vi "CLD 14 Timer Application Solution.vi"() -> ()   [LabVIEW 2009]
doc: "CLD-Lösung 14. Dies ist ein Zustandsautomat in einer Queue. Als Queue wird ein Array verwendet. Der Timer wurde aus CLD-Übung 3 übernommen und angepasst.\n\nDie Timer-FGV läuft immer. Als Zeichen dafür, dass der Timer nicht \"aktiv\" ist, wird eine Zielzeit gleich null verwendet."
uses:
  CLD 14 State Machine Enum.ctl
  CLD 14 CSV file enum.ctl
  CLD 14 FGV Enum.ctl
panel:
  out "Zielzeit (s)":dbl
  out "Verstrichene Zeit (s)":dbl format="%#.2g"
  in  "Stopp":bool
  in  "Anhalten":bool
  in  "Abbrechen":bool
  in  "Starten":bool
  in  "Fehler (Eingang)":errorcluster
  out "Fehler (Ausgang)":errorcluster
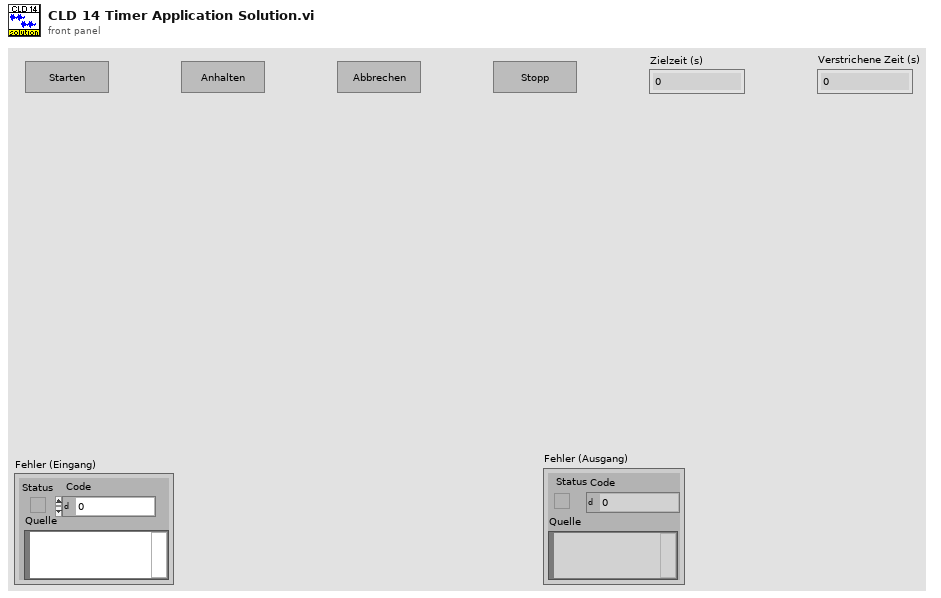
[diagram p1: front panel]
types:
  T1 = typedef "CLD 14 FGV Enum.ctl" = enum16{"Timer starten", "Zeit lesen", "Anhalten", "Fortsetzen"}
  T2 = typedef "CLD 14 State Machine Enum.ctl" = enum16{"Ruhezustand", "Initialisieren", "Zustand ausführen", "Zeit ändern", "Zeit prüfen", "Startzeit", "Anhalten", "Fortsetzen"}
  T3 = cluster{"Status":bool, "Code":i32, "Quelle":string}
  T4 = typedef "CLD 14 CSV file enum.ctl" = enum16{"CSV lesen", "CSV schreiben"}
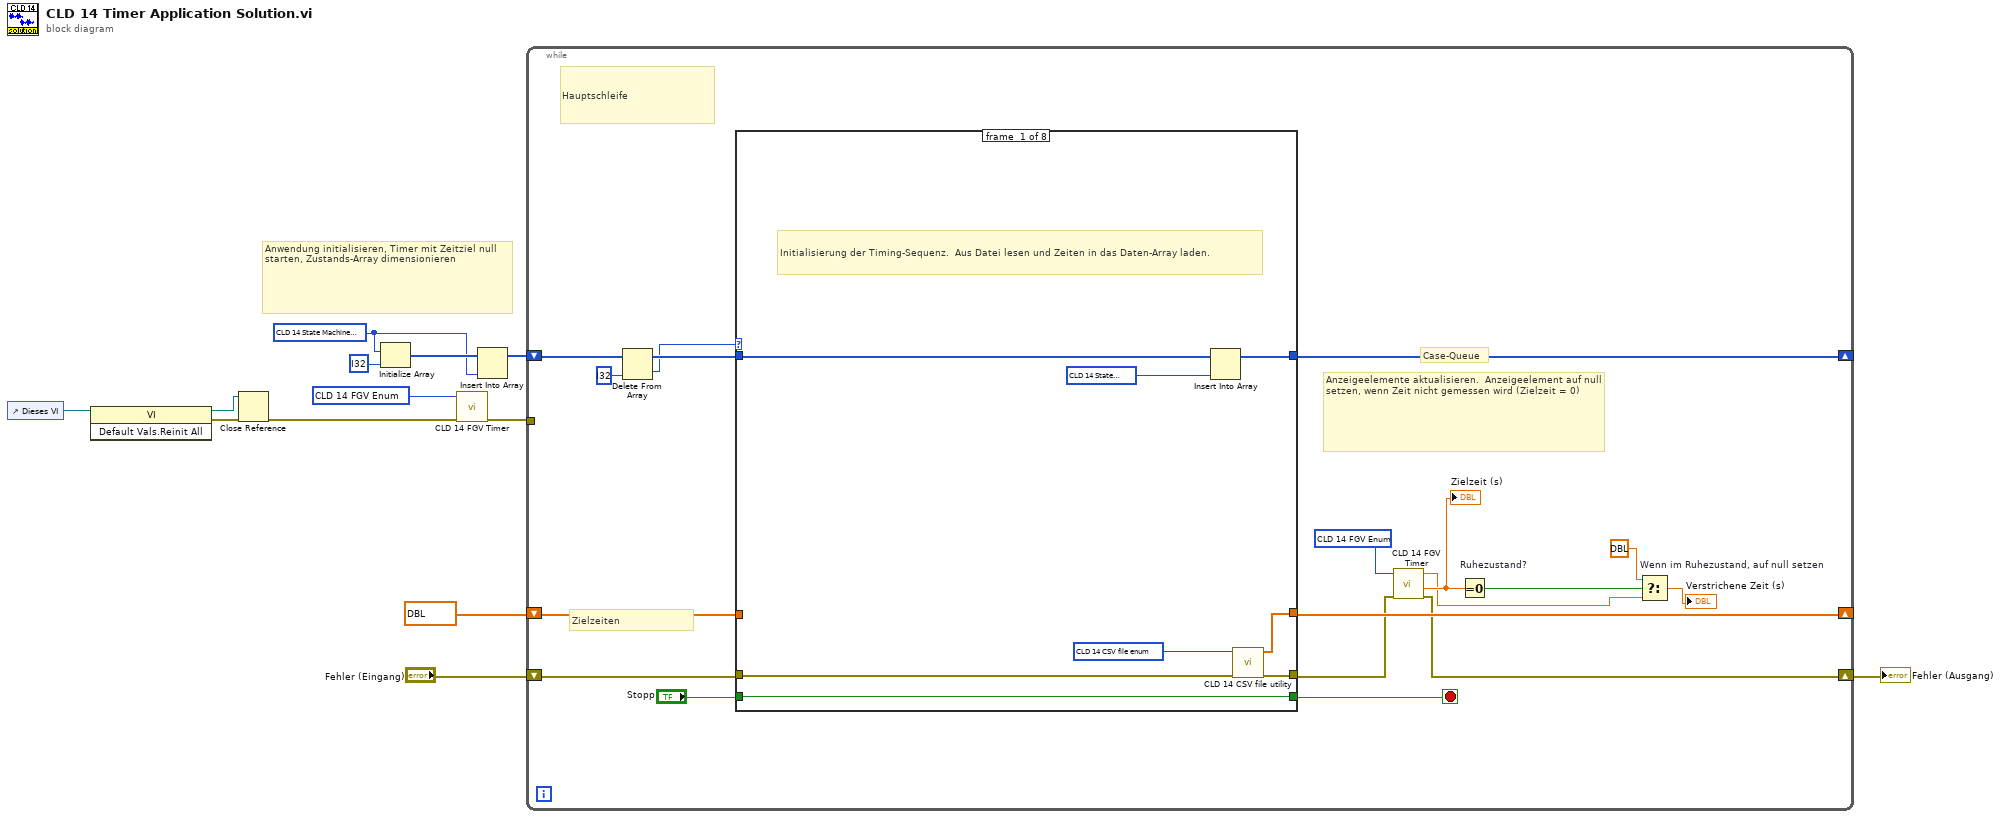
[diagram p0: block diagram]
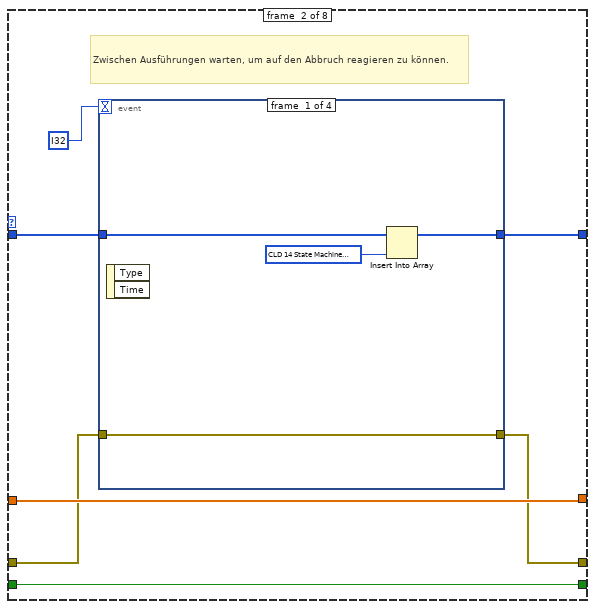
[diagram p2: hidden frame]
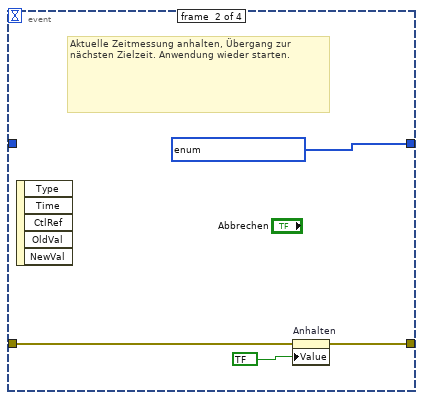
[diagram p3: hidden frame]
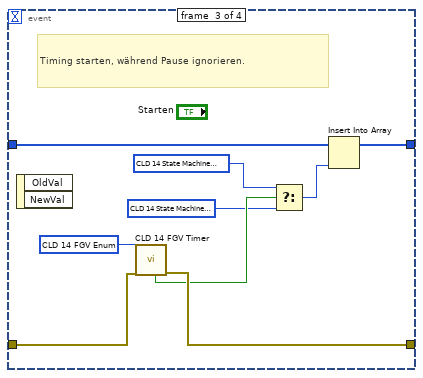
[diagram p4: hidden frame]
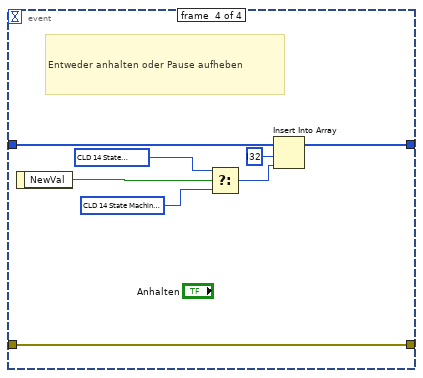
[diagram p5: hidden frame]
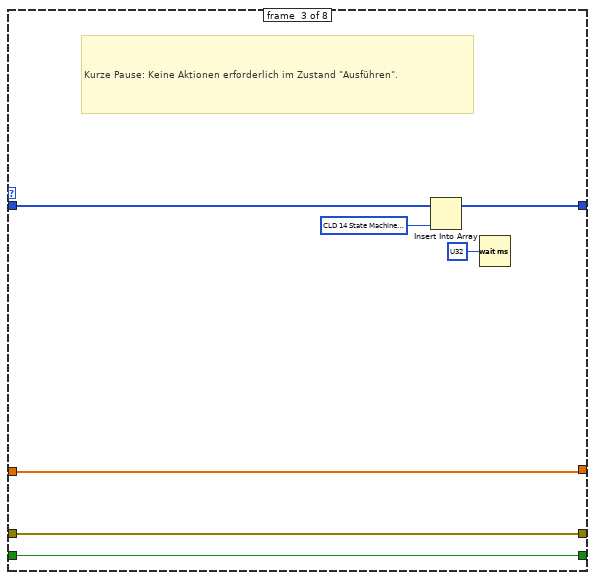
[diagram p6: hidden frame]
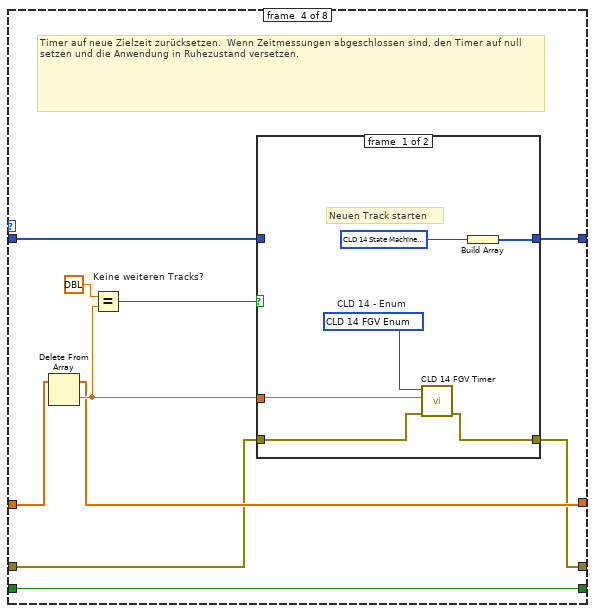
[diagram p7: hidden frame]
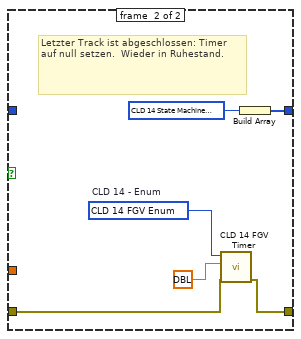
[diagram p8: hidden frame]
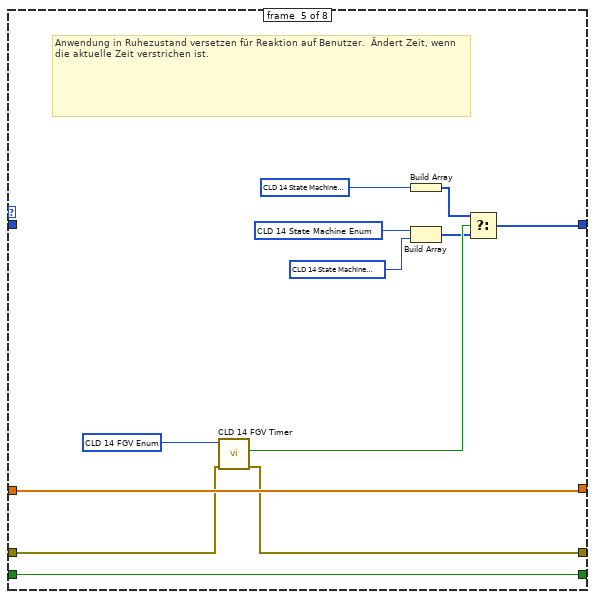
[diagram p9: hidden frame]
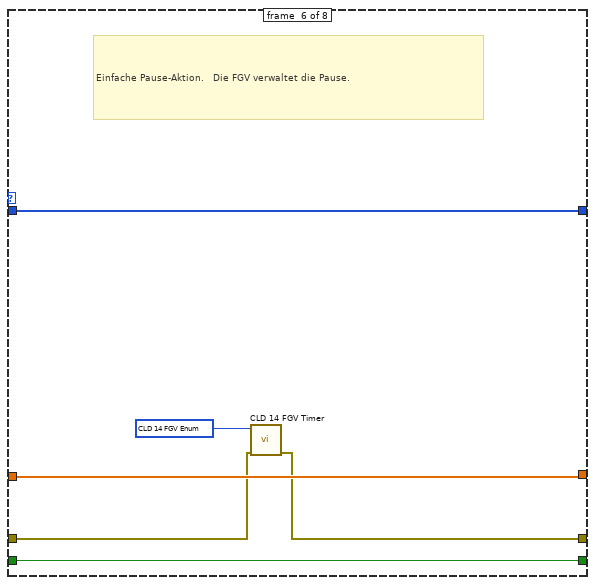
[diagram p10: hidden frame]
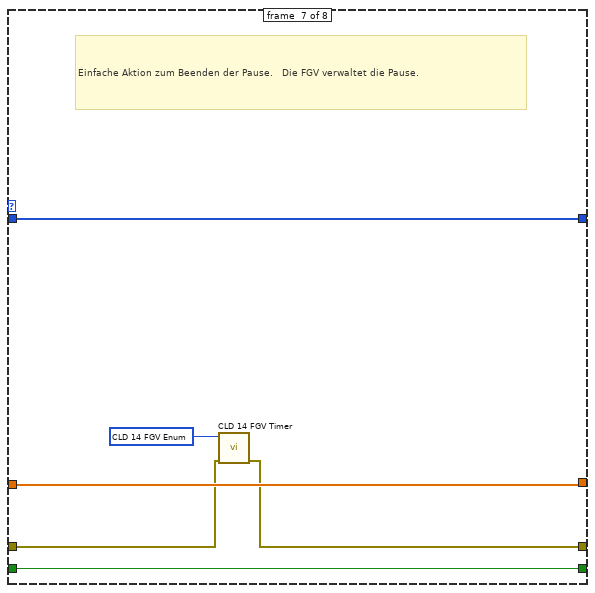
[diagram p11: hidden frame]
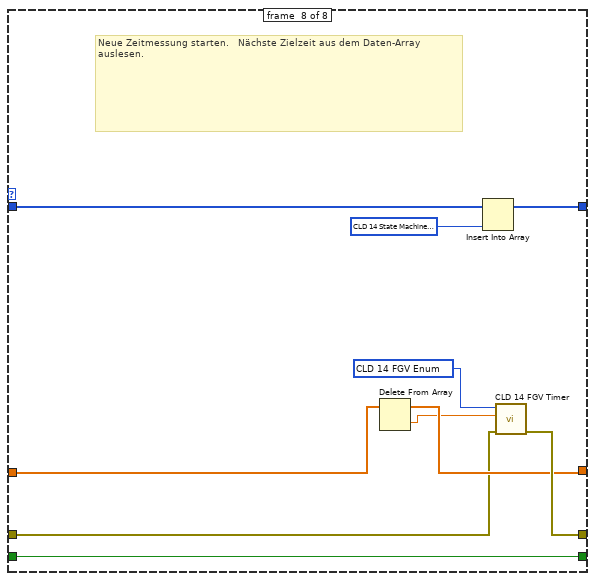
[diagram p12: hidden frame]
diagram:
  w2 = T2 ? ("CLD 14")
  # "Anwendung initialisieren, Timer mit Zeitziel null starten, Zustands-Array dimensionieren"
  n1 = control-ref of="Dieses VI"() -> (w8:refnum<vi>)
  n2 = invoke on="Invoke Node" class="VI" method="Default Vals.Reinit All"(reference=w8) -> (reference out=w9:refnum<vi>, error out=w10:errorcluster)  [unwired: 2 in, 1 out]
  n3 = Close Reference(reference=w9, error in (no error)=w10) -> (error out=w7:errorcluster)
  n4 = Initialize Array(w2, i32 ? ("Dimension")) -> (w4:T2[])
  n5 = call "CLD 14 FGV Timer.vi"("Fehler (Eingang)"=w7, "CLD 14 - FGV-Enum"=T1 ?) -> ("Fehler (Ausgang)"=w6:T3)  [unwired: 5 in, 4 out]
  n6 = Insert Into Array(array=w4, new element=w2) -> (w3:T2[])  [unwired: 1 in]
  n7 = while {
    shift-right: [w31] -> _
    shift-left: w3 -> [w24]
    shift-right: [w26] -> _
    shift-left: dbl[] ? ("Array") -> [w29]
    tunnel: w6 -> [_]
    shift-right: [w14] -> w12
    shift-left: "Fehler (Eingang)" -> [w30]
    stop <- w28 stop-if-true
    # "Case-Queue"
    # "Zielzeiten"
    # "Anzeigeelemente aktualisieren.  Anzeigeelement auf null setzen, wenn Zeit nicht gemessen wird (Zielzeit = 0)"
    # "Hauptschleife"
    n8 = Delete From Array(array=w24, index=i32 ? ("Index")) -> (deleted portion=w23:T2, array with subset deleted=w25:T2[])  [unwired: 1 in]
    n9 = case shown="\"Ruhezustand\", Default" w23 {
      tunnel: [w32 w46 w74 w84 w103 w113 w119 w130] -> w31
      tunnel: w30 -> [w39 w42 w78 w80 w109 w115 w121 w127]
      tunnel: [w38 w41 w78 w79 w108 w114 w120 w133] -> w15
      tunnel: [w36 w43 w76 w82 w112 w118 w124 w131] -> w26
      tunnel: w29 -> [_ w43 w76 w83 w112 w118 w124 w132]
      tunnel: "Stopp" -> [w35 w45 w77 w88 w111 w117 w123 w134]
      tunnel: [w35 w45 w77 w88 w111 w117 w123 w134] -> w28
      tunnel: w25 -> [w33 w40 w72 w81 _ w113 w119 w128]
      frame #0 {
        # "Initialisierung der Timing-Sequenz.  Aus Datei lesen und Zeiten in das Daten-Array laden."
        n10 = Insert Into Array(array=w33, new element=T2 ? ("CLD 14")) -> (w32:T2[])  [unwired: 1 in]
        n11 = call "CLD 14 CSV file utility.vi"("Fehler (Eingang)"=w39, "CLD 14 - Timer-Enum"=T4 ? ("Enum für Timer 1 in CLD 8")) -> ("Fehler (Ausgang)"=w38:T3, "Array"=w36:dbl[])  [unwired: 8 in]
      }
      frame #1 {
        # "Zwischen Ausführungen warten, um auf den Abbruch reagieren zu können."
        n12 = event shown="[1] \"Abbrechen\": Value Change" {
          selector: _ -> [_ _ _ _]
          dyn-events: _ -> [_ _ _ _]
          timeout: i32 ? -> [_ _ _ _]
          tunnel: [w49 w54 w63 w69] -> w46
          tunnel: [w50 w51 w59 w71] -> w41
          tunnel: w42 -> [w50 w52 w60 w71]
          tunnel: w40 -> [w47 _ w62 w70]
          event #0 {
            n13 = event-data() -> ()  [unwired: 1 in, 2 out]
            n14 = Insert Into Array(array=w47, new element=T2 ? ("CLD 14")) -> (w49:T2[])  [unwired: 1 in]
          }
          event #1 {
            w54 = T2[] ? items=["Ruhezustand", "Initialisieren", "Zustand ausführen", "Zeit ändern", "Zeit prüfen", "Startzeit", "Anhalten", "Fortsetzen"]
            # "Aktuelle Zeitmessung anhalten, Übergang zur nächsten Zielzeit. Anwendung wieder starten."
            n15 = event-data() -> ()  [unwired: 1 in, 5 out]
            n16 = property on="Anhalten" class="Bool (strict)"(error in=w52, "Value"=bool ? ("Anhalten")) -> (error out=w51:errorcluster)  [unwired: 1 in, 1 out]
          }
          event #2 {
            # "Timing starten, während Pause ignorieren."
            n17 = event-data() -> ()  [unwired: 1 in, 2 out]
            n18 = call "CLD 14 FGV Timer.vi"("Fehler (Eingang)"=w60, "CLD 14 - FGV-Enum"=T1 ? ("CLD 14 - Enum")) -> ("Fehler (Ausgang)"=w59:T3, "Anhalten?"=w58:bool)  [unwired: 5 in, 3 out]
            n19 = Select(t=T2 ? ("CLD 14"), s=w58, f=T2 ? ("CLD 14")) -> (s? t:f=w55:T2)
            n20 = Insert Into Array(array=w62, new element=w55) -> (w63:T2[])  [unwired: 1 in]
          }
          event #3 {
            # "Entweder anhalten oder Pause aufheben"
            n21 = event-data() -> ("NewVal"=w68:bool)  [unwired: 1 in]
            n22 = Select(t=T2 ? ("Neues Element/Teil-Array"), s=w68, f=T2 ? ("Neues Element/Teil-Array")) -> (s? t:f=w65:T2)
            n23 = Insert Into Array(array=w70, index=i32 ? ("Index"), new element=w65) -> (w69:T2[])
          }
        }
      }
      frame #2 {
        # "Kurze Pause: Keine Aktionen erforderlich im Zustand \"Ausführen\"."
        n24 = Insert Into Array(array=w72, new element=T2 ? ("CLD 14")) -> (w74:T2[])  [unwired: 1 in]
        n25 = Wait (ms)(milliseconds to wait=u32 ? ("Zu wartende ms")) -> ()  [unwired: 1 out]
      }
      frame #3 {
        # "Timer auf neue Zielzeit zurücksetzen.  Wenn Zeitmessungen abgeschlossen sind, den Timer auf null setzen und die Anwendung in Ruhezustand versetzen."
        n26 = Delete From Array(array=w83) -> (deleted portion=w85:dbl, array with subset deleted=w82:dbl[])  [unwired: 2 in]
        n27 = Equal? "Keine weiteren Tracks?"(x=dbl ?, y=w85) -> (x = y?=w86:bool)
        n28 = case shown="True" w86 {
          tunnel: w85 -> [w94 _]
          tunnel: w80 -> [w93 w98]
          tunnel: [w89 w95] -> w84
          tunnel: w81 -> [_ _]
          tunnel: [w91 w97] -> w79
          frame #0 {
            w92 = T1 ?  # CLD 14 - Enum
            # "Neuen Track starten"
            n29 = call "CLD 14 FGV Timer.vi"("Fehler (Eingang)"=w93, "Zielzeit (s) [0]"=w94, "CLD 14 - FGV-Enum"=w92) -> ("Fehler (Ausgang)"=w91:T3)  [unwired: 4 in, 4 out]
            n30 = Build Array(T2 ? ("CLD 14")) -> (w89:T2[])
          }
          frame #1 {
            w100 = T1 ?  # CLD 14 - Enum
            # "Letzter Track ist abgeschlossen: Timer auf null setzen.  Wieder in Ruhestand."
            n31 = call "CLD 14 FGV Timer.vi"("Fehler (Eingang)"=w98, "Zielzeit (s) [0]"=dbl ? ("Zielzeit (s)"), "CLD 14 - FGV-Enum"=w100) -> ("Fehler (Ausgang)"=w97:T3)  [unwired: 4 in, 4 out]
            n32 = Build Array(T2 ? ("CLD 14")) -> (w95:T2[])
          }
        }
      }
      frame #4 {
        # "Anwendung in Ruhezustand versetzen für Reaktion auf Benutzer.  Ändert Zeit, wenn die aktuelle Zeit verstrichen ist."
        n33 = call "CLD 14 FGV Timer.vi"("Fehler (Eingang)"=w109, "CLD 14 - FGV-Enum"=T1 ? ("CLD 14 - Enum")) -> ("Fehler (Ausgang)"=w108:T3, "Ist Zeit verstrichen?"=w107:bool)  [unwired: 5 in, 3 out]
        n34 = Build Array(T2 ? ("CLD 14")) -> (w105:T2[])
        n35 = Build Array(T2 ? ("CLD 14"), T2 ? ("CLD 14")) -> (w104:T2[])
        n36 = Select(t=w105, s=w107, f=w104) -> (s? t:f=w103:T2[])
      }
      frame #5 {
        # "Einfache Pause-Aktion.   Die FGV verwaltet die Pause."
        n37 = call "CLD 14 FGV Timer.vi"("Fehler (Eingang)"=w115, "CLD 14 - FGV-Enum"=T1 ? ("CLD 14 - Enum")) -> ("Fehler (Ausgang)"=w114:T3)  [unwired: 5 in, 4 out]
      }
      frame #6 {
        # "Einfache Aktion zum Beenden der Pause.   Die FGV verwaltet die Pause."
        n38 = call "CLD 14 FGV Timer.vi"("Fehler (Eingang)"=w121, "CLD 14 - FGV-Enum"=T1 ? ("CLD 14 - Enum")) -> ("Fehler (Ausgang)"=w120:T3)  [unwired: 5 in, 4 out]
      }
      frame #7 {
        # "Neue Zeitmessung starten.   Nächste Zielzeit aus dem Daten-Array auslesen."
        n39 = Delete From Array(array=w132) -> (deleted portion=w126:dbl, array with subset deleted=w131:dbl[])  [unwired: 2 in]
        n40 = Insert Into Array(array=w128, new element=T2 ? ("CLD 14")) -> (w130:T2[])  [unwired: 1 in]
        n41 = call "CLD 14 FGV Timer.vi"("Fehler (Eingang)"=w127, "Zielzeit (s) [0]"=w126, "CLD 14 - FGV-Enum"=T1 ? ("CLD 14 - Enum")) -> ("Fehler (Ausgang)"=w133:T3)  [unwired: 4 in, 4 out]
      }
    }
    n42 = call "CLD 14 FGV Timer.vi"("Fehler (Eingang)"=w15, "CLD 14 - FGV-Enum"=T1 ? ("CLD 14 - Enum")) -> ("Fehler (Ausgang)"=w14:T3, "Zielzeit (Ausgang)"=w19:dbl, "Verstrichene Zeit (s,ms)"=w17:dbl)  [unwired: 5 in, 2 out]
    "Zielzeit (s)" <- w19
    n43 = Equal To 0? "Ruhezustand?"(x=w19) -> (x = 0?=w20:bool)
    n44 = Select "Wenn im Ruhezustand, auf null setzen"(t=dbl ?, s=w20, f=w17) -> (s? t:f=→"Verstrichene Zeit (s)":dbl)
  }
  "Fehler (Ausgang)" <- w12
